vi "temp_to_volt.vi"(2 "Temperatura °C":dbl, 3 "Manual/Automatico":bool) -> (0 "Temperatura aleatoria °c":dbl, 1 "Voltaje":dbl format="%f Voltios")   [LabVIEW 2018]
doc: "Esta función apartir de una Temperatura ingresada por el usuario emula a su salida el Voltaje de un MCP9701A"
panel:
  # "https://www.microchip.com/wwwproducts/en/MCP9701A"
  # "Sensor MCP9701A"
  # "Temp. Range (°C)\n-40 to a125"
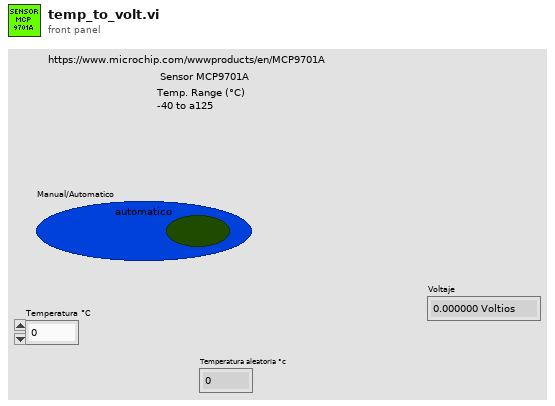
[diagram p1: front panel]
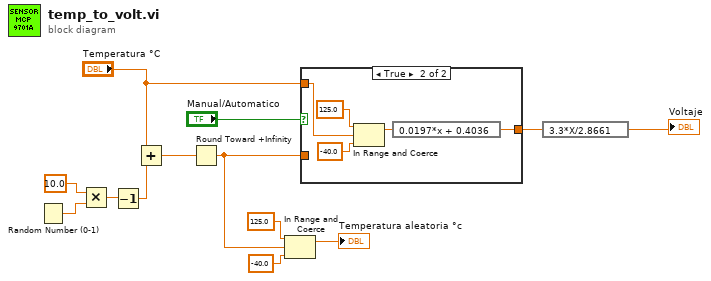
[diagram p0: block diagram]
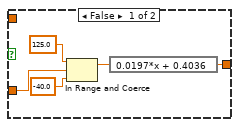
[diagram p2: hidden frame]
diagram:
  n1 = Random Number (0-1)() -> (number: 0 to 1=w13:dbl)
  n2 = Multiply(x=10.0, y=w13) -> (x*y=w8:dbl)
  n3 = Decrement(x=w8) -> (x-1=w7:dbl)
  n4 = Add(x="Temperatura °C", y=w7) -> (x+y=w11:dbl)
  n5 = Round Toward +Infinity(x=w11) -> (ceil(x): smallest int >= x=w2:dbl)
  n6 = In Range and Coerce(upper limit=125.0, x=w2, lower limit=-40.0) -> (coerced(x)=→"Temperatura aleatoria °c":dbl)  [unwired: 1 out]
  n7 = case shown="True" "Manual/Automatico" {
    tunnel: [w18 w23] -> w6
    tunnel: "Temperatura °C" -> [_ w19]
    tunnel: w2 -> [w15 _]
    frame False {
      n8 = In Range and Coerce(upper limit=125.0, x=w15, lower limit=-40.0) -> (coerced(x)=w14:dbl)  [unwired: 1 out]
      n9 = expression code="0.0197*x + 0.4036"(w14) -> (w18:dbl)
    }
    frame True {
      n10 = In Range and Coerce(upper limit=125.0, x=w19, lower limit=-40.0) -> (coerced(x)=w22:dbl)  [unwired: 1 out]
      n11 = expression code="0.0197*x + 0.4036"(w22) -> (w23:dbl)
    }
  }
  n12 = expression code="3.3*X/2.8661"(w6) -> (→"Voltaje":dbl)
